vi "Sub_std_dev_update.vi"(6 "Frequency differentials":dbl[](array[numeric]), 10 "standard dev":bool, 11 "Setup Parameters":T1) -> (3 "Setup Parameters":T1)   [LabVIEW 2021]
uses:
  <vilib>/Analysis/NI_AALBase.lvlib
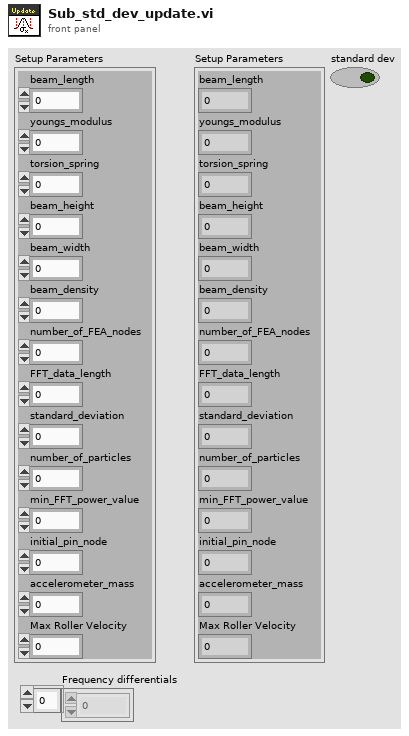
[diagram p1: front panel]
types:
  T1 = cluster{"beam_length":dbl, "youngs_modulus":dbl, "torsion_spring":dbl, "beam_height":dbl, "beam_width":dbl, "beam_density":dbl, "number_of_FEA_nodes":i32, "FFT_data_length":i32, "standard_deviation":dbl, "number_of_particles":i32, "min_FFT_power_value":dbl, "initial_pin_node":i32, "accelerometer_mass":dbl, "Max Roller Velocity":dbl}
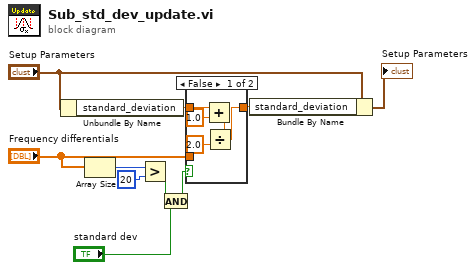
[diagram p0: block diagram]
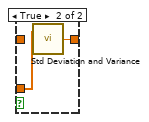
[diagram p2: hidden frame]
diagram:
  n1 = Unbundle By Name("Setup Parameters") -> ("standard_deviation"=w7:dbl)
  n2 = Array Size(array="Frequency differentials") -> (size(s)=w9:i32)
  n3 = Greater?(x=w9, y=20) -> (0:w3:bool)
  n4 = And(x="standard dev", y=w3) -> (x .and. y?=w2:bool)
  n5 = case shown="False" w2 {
    tunnel: w7 -> [w13 _]
    tunnel: [w12 w16] -> w6
    tunnel: "Frequency differentials" -> [_ w17]
    frame False {
      n6 = Add(x=w13, y=1.0) -> (x+y=w14:dbl)
      n7 = Divide(x=w14, y=2.0) -> (x/y=w12:dbl)
    }
    frame True {
      n8 = call <vilib>:"Std Deviation and Variance.vi"("X"=w17) -> ("standard deviation"=w16:dbl)  [unwired: 1 in, 2 out]
    }
  }
  n9 = Bundle By Name(cluster="Setup Parameters", "standard_deviation"=w6) -> (→"Setup Parameters":T1)
